vi "ADStar Navigation - Known Map.vi"() -> ()   [LabVIEW 2013]
doc: "This example continually replans a path from Start to Goal while following the best known path, including through obstacles if necessary.\nThe Anytime D* search algorithm is useful when the world or the robot's understanding of the world is changing. Anytime D* maintains more information than the A* search algorithm so the robot can backtrack and find a new path more easily if it discovers the original path will not work."
uses:
  <vilib>/robotics/Navigation/shared/WorldMap/OccupancyGridWorldMap/NI_Robotics_OccupancyGridWorldMap.lvclass
  <vilib>/robotics/Navigation/Anytime D Star/NI_Robotics_AnytimeDStar.lvclass
panel:
  in  "Random Obstacles?":bool
  in  "Step Through":bool
  in  "% Random Obstacles":dbl=40.0 min=0.0 max=100.0 step=1.0 format="%#_3g"
  in  "goal y":i32=35
  in  "goal x":i32=50
  out "Open List Size":i32(graph)=1665
  out "path on obstacles":dbl[][](graph)
  out "AD* Open Nodes":i32=1665 caption="size"
  out "Path Cost":dbl(graph)
  in  "Epsilon":i32=2 min=1
  out "AD* Path Cost":dbl caption="path cost"
  in  "y start":i32
  in  "x start":i32
  in  "Move Robot":i32=1 min=0
  in  "Overhaul":i32=25
  in  "step button":bool
  out "AD* Time":u32=117 caption="seconds"
  out "Compute Path Time":u32(graph)=117
  in  "stop":bool
  # "The Anytime D* search algorithm is useful when the world or the robot's understanding of the world is changing.  Anytime D* maintains more information\n than the A* search algorithm so the robot can backtrack and find a new path more easily if it discovers the original path will not work."
  # "This example continually replans a path from Start to Goal while \nfollowing the best known path, including through obstacles if necessary."
  # "Configuration"
  # "X"
  # "Y"
  # "Start"
  # "Goal"
  # "Run Mode"
  # "Run-time Control"
  # "Detection radius of robot's sensors."
  # "Number of steps the robot takes after each plan."
  # "Number of steps before AD* plans from scratch."
  # "1) Choose the Start and Goal location and the % Random Obstacles.\n2) Run the VI.\n3) Adjust the controls in the Run-time Controls section to see the \n     effect each option has on path planning\n4) Change the Run Mode to Single Step to pause after each time\n the AD* VI runs"
  # "A higher epsilon results in a faster but less optimal search."
  # "Continuous"
  # "Single Step"
  # "Robot"
  # "Obstacle"
  # "Unknown"
  # "Free"
  # "Path"
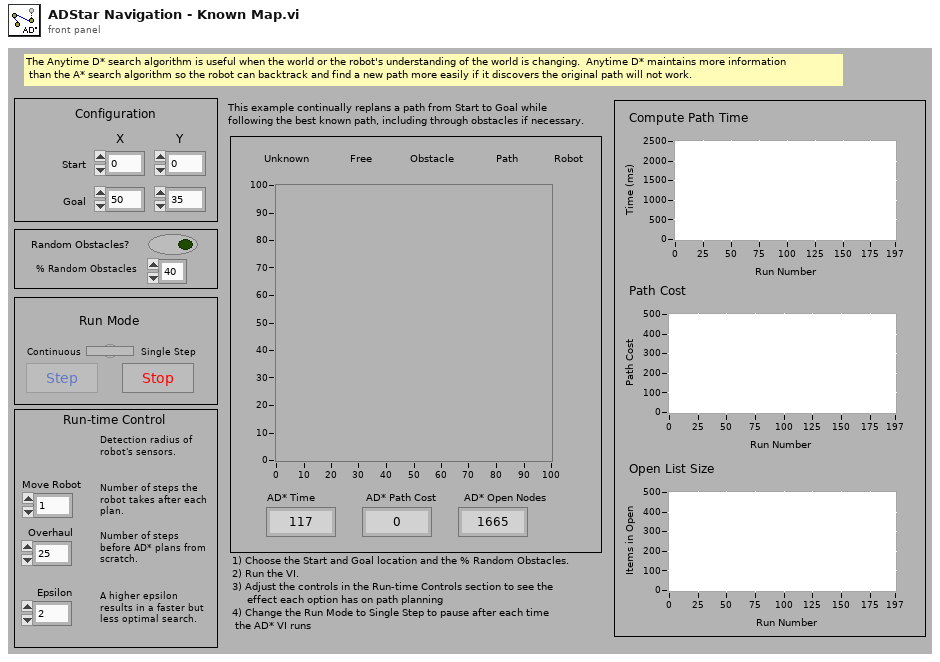
[diagram p1: front panel]
types:
  T1 = enum8{"Enabled", "Disabled", "Disabled and Grayed Out"}
  T2 = cluster{"epsilon":dbl, "run number":i32, "open list size":i32}
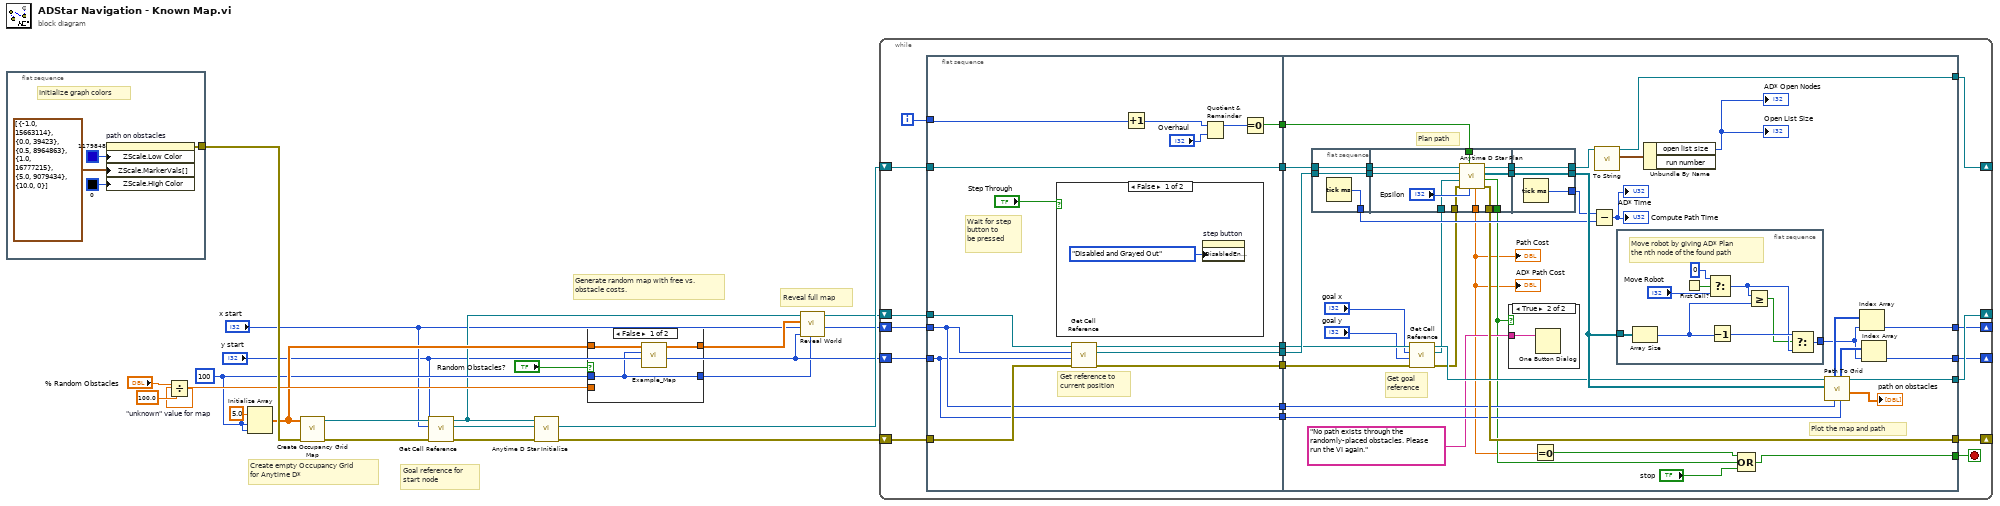
[diagram p0: block diagram]
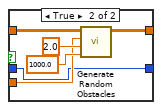
[diagram p2: hidden frame]
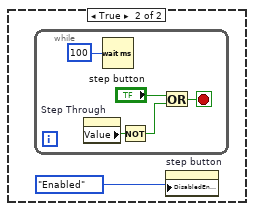
[diagram p3: hidden frame]
diagram:
  w8 = 100 ("dimension size")
  w19 = 5.0  # "unknown" value for map
  # "Reveal full map"
  # "Goal reference for\nstart node"
  # "Generate random map with free vs.\nobstacle costs."
  # "Create empty Occupancy Grid\nfor Anytime D*"
  n1 = flat-sequence {
    tunnel: [w21] -> w13
    frame #0 {
      # "Initialize graph colors"
      n2 = property on="path on obstacles" class="IntGraph (strict)"("ZScale.Low Color"=u32 1179848, "ZScale.MarkerVals[]"=cluster{dbl, u32}[] [{-1.0, 15663114}, {0.0, 39423}, {0.5, 8964863}, {1.0, 16777215}, {5.0, 9079434}, {10.0, 0}], "ZScale.High Color"=u32 0) -> (error out=w21:errorcluster)  [unwired: 2 in, 1 out]
    }
  }
  n3 = Divide(x="% Random Obstacles", y=100.0) -> (x/y=w10:dbl)
  n4 = Initialize Array(w19, w8, w8) -> (w9:dbl[][])
  n5 = call <vilib>:"Create Occupancy Grid Map.vi"("error in (no error)"=w13, "occupancy grid"=w9) -> ("error out"=w16:errorcluster, "map reference out"=w17:refnum<data-value>)  [unwired: 8 in]
  n6 = call <vilib>:"Get Cell Reference.vi"("error in (no error)"=w16, "y"="y start", "x"="x start", "map reference in"=w17) -> ("error out"=w15:errorcluster, "cell reference"=w18:refnum<data-value>, "map reference out"=w6:refnum<data-value>)  [unwired: 4 in, 1 out]
  n7 = call <vilib>:"Anytime D Star Initialize.vi"("error in (no error)"=w15, "start reference"=w18, "map reference in"=w6) -> ("error out"=w14:errorcluster, "Anytime D*"=w12:refnum<class "NI_Robotics_AnytimeDStar.lvclass">)  [unwired: 7 in]
  n8 = case shown="False" "Random Obstacles?" {
    tunnel: w10 -> [_ w31]
    tunnel: w9 -> [w27 w30]
    tunnel: [w26 w29] -> w4
    tunnel: w8 -> [w25 w28]
    tunnel: [w25 w28] -> w1
    frame False {
      n9 = call "Example_Map.vi"("dimension size"=w25, "Array in"=w27) -> ("Array out"=w26:dbl[][])  [unwired: 9 in]
    }
    frame True {
      n10 = call "Generate Random Obstacles.vi"("obstacle cost"=1000.0, "free cost"=2.0, "chance"=w31, "cost in"=w30) -> ("cost out"=w29:dbl[][])  [unwired: 7 in]
    }
  }
  n11 = call "Reveal World.vi"("radius"=w1, "y"="y start", "x"="x start", "cost in"=w4, "map reference in"=w6) -> ("map reference in 2"=w5:refnum<data-value>)  [unwired: 5 in, 1 out]
  n12 = while {
    shift-right: [w43] -> _
    shift-left: w12 -> [w52]
    shift-right: [w50] -> _
    shift-left: w5 -> [w51]
    shift-right: [w42] -> _
    shift-left: "x start" -> [w45]
    shift-right: [w41] -> _
    shift-left: "y start" -> [w44]
    shift-right: [w36] -> _
    shift-left: w14 -> [w38]
    i -> [w40]
    stop <- w49 stop-if-true
    n13 = flat-sequence {
      tunnel: w40 -> [w59]
      tunnel: w51 -> [w53]
      tunnel: w52 -> [w66]
      tunnel: [w66] -> w48
      tunnel: [w65] -> w47
      tunnel: [w64] -> w46
      tunnel: w45 -> [w55]
      tunnel: w44 -> [w54]
      tunnel: [w58] -> w39
      tunnel: w38 -> [w57]
      tunnel: [w56] -> w37
      tunnel: [w55] -> w35
      tunnel: [w54] -> w34
      tunnel: [w76] -> w49
      tunnel: [w110] -> w43
      tunnel: [w98] -> w50
      tunnel: [w91] -> w42
      tunnel: [w90] -> w41
      tunnel: w39 -> [w96]
      tunnel: w46 -> [w95]
      tunnel: w47 -> [w89]
      tunnel: w48 -> [w106]
      tunnel: w37 -> [w86]
      tunnel: [w82] -> w36
      tunnel: w35 -> [w81]
      tunnel: w34 -> [w80]
      frame #0 {
        # "Get reference to \ncurrent position"
        # "Wait for step\nbutton to\nbe pressed"
        n14 = case shown="False" "Step Through" {
          frame False {
            n15 = property on="step button" class="Bool (strict)"("DisabledEnum"=T1."Disabled and Grayed Out" ("Disabled")) -> ()  [unwired: 2 in, 2 out]
          }
          frame True {
            n16 = while {
              stop <- w71 stop-if-true
              n17 = property on="Step Through" class="Bool (strict)"() -> ("Value"=w69:bool)  [unwired: 2 in, 2 out]
              n18 = Wait (ms)(milliseconds to wait=u32 100) -> ()  [unwired: 1 out]
              n19 = Not(x=w69) -> (.not. x?=w70:bool)
              n20 = Or(x="step button", y=w70) -> (x .or. y?=w71:bool)
            }
            n21 = property on="step button" class="Bool (strict)"("DisabledEnum"=T1."Enabled" ("Disabled")) -> ()  [unwired: 2 in, 2 out]
          }
        }
        n22 = call <vilib>:"Get Cell Reference.vi"("error in (no error)"=w57, "y"=w54, "x"=w55, "map reference in"=w53) -> ("error out"=w56:errorcluster, "cell reference"=w64:refnum<data-value>, "map reference out"=w65:refnum<data-value>)  [unwired: 4 in, 1 out]
        n23 = Increment(x=w59) -> (x+1=w61:i32)
        n24 = Quotient & Remainder(x=w61, y="Overhaul") -> (x-y*floor(x/y)=w60:i32)  [unwired: 1 out]
        n25 = Equal To 0?(x=w60) -> (x = 0?=w58:bool)
      }
      frame #1 {
        # "Plot the map and path"
        # "Get goal \nreference"
        # "Plan path"
        n26 = flat-sequence {
          tunnel: w106 -> [w123]
          tunnel: w95 -> [w124]
          tunnel: [w124] -> w105
          tunnel: [w123] -> w104
          tunnel: [w122] -> w100
          tunnel: [w131] -> w77
          tunnel: [w130] -> w75
          tunnel: w105 -> [w134]
          tunnel: w104 -> [w135]
          tunnel: [w132] -> w103
          tunnel: [w133] -> w102
          tunnel: w96 -> [w128]
          tunnel: w84 -> [w127]
          tunnel: w83 -> [w126]
          tunnel: [w125] -> w82
          tunnel: [w137] -> w109
          tunnel: [w138] -> w111
          tunnel: w103 -> [w138]
          tunnel: w102 -> [w137]
          tunnel: [w136] -> w101
          frame #0 {
            n27 = Tick Count (ms)() -> (millisecond timer value=w122:u32)
          }
          frame #1 {
            n28 = call <vilib>:"Anytime D Star Plan.vi"("epsilon"="Epsilon", "overhaul (F)"=w128, "error in (no error)"=w126, "new goal reference"=w127, "current reference"=w134, "Anytime D* in"=w135) -> ("error out"=w125:errorcluster, "no valid path exists"=w131:bool, "path references"=w133:refnum<data-value>[], "Anytime D* out"=w132:refnum<class "NI_Robotics_AnytimeDStar.lvclass">, "path cost"=w130:dbl)  [unwired: 1 in]
          }
          frame #2 {
            n29 = Tick Count (ms)() -> (millisecond timer value=w136:u32)
          }
        }
        n30 = call <vilib>:"Get Cell Reference.vi"("error in (no error)"=w86, "y"="goal y", "x"="goal x", "map reference in"=w89) -> ("error out"=w83:errorcluster, "cell reference"=w84:refnum<data-value>, "map reference out"=w85:refnum<data-value>)  [unwired: 4 in, 1 out]
        n31 = case shown="True" w77 {
          tunnel: "No path exists through the randomly-placed obstacles. Please run the VI again." -> [_ w112]
          frame False {
          }
          frame True {
            n32 = One Button Dialog(message=w112) -> ()  [unwired: 1 in, 1 out]
          }
        }
        n33 = Equal To 0?(x=w75) -> (x = 0?=w74:bool)
        n34 = Subtract(x=w101, y=w100) -> (x-y=→"Compute Path Time" →"AD* Time":u32)
        n35 = call <vilib>:"To String.vi"("Anytime D* in"=w111) -> ("output"=w108:T2, "Anytime D* out"=w110:refnum<class "NI_Robotics_AnytimeDStar.lvclass">)  [unwired: 8 in, 1 out]
        n36 = flat-sequence {
          tunnel: w109 -> [w120]
          tunnel: [w113] -> w92
          frame #0 {
            # "Move robot by giving AD* Plan\nthe nth node of the found path"
            n37 = Array Size(array=w120) -> (size(s)=w117:i32)
            n38 = First Call?() -> (First Call?: T/F=w119:bool)
            n39 = Select(t=0, s=w119, f="Move Robot") -> (s? t:f=w116:i32)
            n40 = Decrement(x=w117) -> (x-1=w121:i32)
            n41 = Greater Or Equal?(x=w116, y=w117) -> (x >= y?=w115:bool)
            n42 = Select(t=w121, s=w115, f=w116) -> (s? t:f=w113:i32)
          }
        }
        n43 = Unbundle By Name(w108) -> ("open list size"=→"Open List Size" →"AD* Open Nodes":i32)  [unwired: 1 out]
        n44 = Compound Arithmetic op=OR(w74, w77, "stop") -> (w76:bool)
        n45 = call "Path To Grid.vi"("current y"=w80, "current x"=w81, "path references"=w109, "map reference in"=w85) -> ("path on obstacles"=→"path on obstacles":dbl[][], "map reference out"=w98:refnum<data-value>, "y coordinates"=w94:i32[], "x coordinates"=w93:i32[])  [unwired: 3 in, 1 out]
        n46 = Index Array(array=w93, index=w92) -> (element=w91:i32)
        n47 = Index Array(array=w94, index=w92) -> (element=w90:i32)
        "AD* Path Cost" <- w75
        "Path Cost" <- w75
      }
    }
  }
